vi "Get GUI reference.vi"(8 "error in (no error)":errorcluster, 11 "Schedule Block in":refnum<class "Schedule Block.lvclass">) -> (0 "error out":errorcluster, 2 "This VI":refnum<vi>, 3 "Schedule Block out":refnum<class "Schedule Block.lvclass">)   [LabVIEW 2020, in "TALOS.lvlib" / "Run Utilities.lvlib" / "Schedule Block.lvclass"]
doc: "Create a GUI element for this SBlock"
uses:
  Schedule Block.lvclass
  Schedule Block.lvclass/Schedule Block.ctl
panel:
  out "Kasli":string
  out "Common Parameters":string[][](array[string])
  out "Number of repetitions":u16=1 min=1
  out "Script name":string
  # "Parameter Name"
  # "Parameter Value"
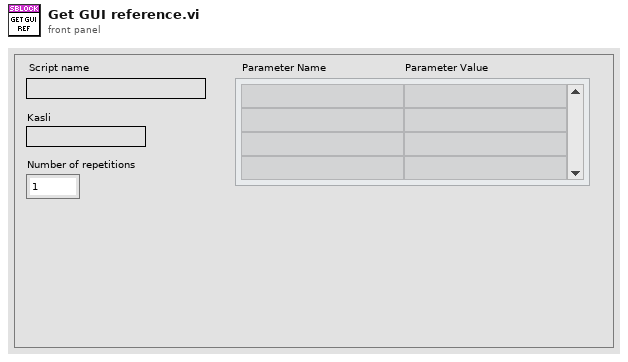
[diagram p1: front panel]
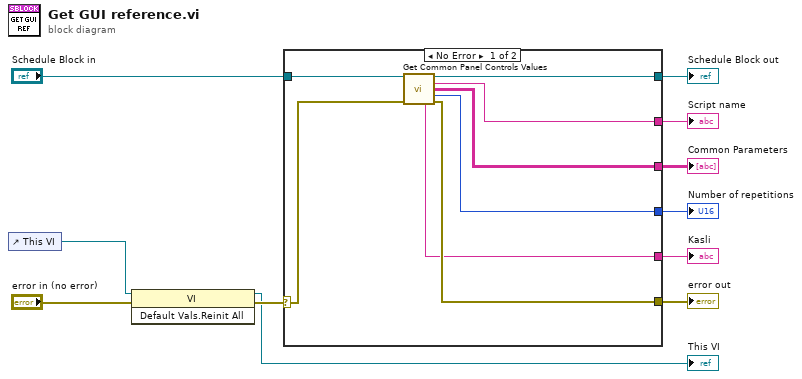
[diagram p0: block diagram]
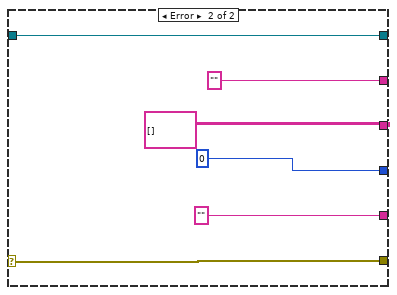
[diagram p2: hidden frame]
diagram:
  n1 = control-ref of="This VI"() -> (w2:refnum<vi>)
  n2 = invoke class="VI" method="Default Vals.Reinit All"(reference=w2, error in="error in (no error)") -> (reference out=→"This VI":refnum<vi>, error out=w4:errorcluster)  [unwired: 1 in, 1 out]
  n3 = case shown="No Error" w4 {
    selector: w4 -> [w17 w25]
    tunnel: [w16 w25] -> w11
    tunnel: [w18 w24] -> w9
    tunnel: "Schedule Block in" -> [w19 w24]
    tunnel: [w12 u16 0 ("Number of repetitions")] -> w8
    tunnel: [w14 "" ("name")] -> w7
    tunnel: [w15 string[][] [] ("Common Parameters")] -> w6
    tunnel: [w13 ""] -> w5
    frame No Error {
      n4 = call-dynamic "Get Common Panel Controls Values.vi"("Schedule Block in"=w19, "error in (no error)"=w17) -> ("Schedule Block out"=w18:refnum<class "Schedule Block.lvclass">, "Script Name"=w14:string, "Common Parameters"=w15:string[][], "Number of repetitions"=w12:u16, "FPGA Name"=w13:string, "error out"=w16:errorcluster)  [unwired: 7 in, 1 out]
    }
    frame Error {
    }
  }
  "error out" <- w11
  "Schedule Block out" <- w9
  "Common Parameters" <- w6
  "Script name" <- w7
  "Number of repetitions" <- w8
  "Kasli" <- w5
